vi "Stop Core.vi"(10 "final error code":i32, 11 "MQTT-Server in":refnum<class "MQTT-Server.lvclass">) -> (3 "MQTT-Server out":refnum<class "MQTT-Server.lvclass">)   [LabVIEW 2023, in "MQTT-Server.lvlib" / "MQTT-Server.lvclass"]
doc: "(<B>Filename</B>: Actor Framework.lvlib:Actor.lvclass:Stop Core.vi)\n\nDefines what the actor does before it stops. Use the <B>final error code</B> input to determine whether the actor shut down in response to an error.\n\nBy default, this method passes the Stop message along to all auto-stop nested actors. A descendant class may override this method to define additional behavior, such as shutting down any processes the actor initiated in its override of the Actor Core method."
uses:
  MQTT-Server.lvclass
  MQTT-Server.lvclass/MQTT-Server.ctl
  <vilib>/ActorFramework/Actor/Actor.lvclass
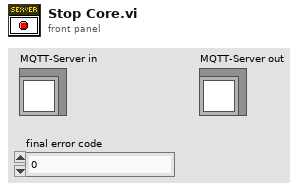
[diagram p1: front panel]
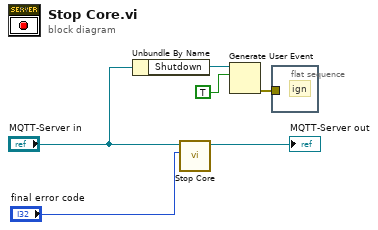
[diagram p0: block diagram]
diagram:
  n1 = Unbundle By Name("MQTT-Server in") -> ("Shutdown"=w3:refnum<user-event>)
  n2 = call-parent "Stop Core.vi"("final error code"="final error code", "Actor in"="MQTT-Server in") -> ("Actor out"=→"MQTT-Server out":refnum<class "MQTT-Server.lvclass">)  [unwired: 9 in]
  n3 = Generate User Event(user event=w3, event data cluster=TRUE ("event data")) -> (error out=w1:errorcluster)  [unwired: 2 in, 1 out]
  n4 = flat-sequence {
    tunnel: w1 -> [_]
    frame #0 {
      # "ign"
    }
  }
